vi "DAQ with LabVIEW 2.0.vi"() -> ()   [LabVIEW 2020]
uses:
  <vilib>/MakerHub/LINX/Public/Peripherals/Analog/Analog Read 1 Chan.vi
  <vilib>/MakerHub/LINX/Public/Peripherals/Digital/Digital Write 1 Chan.vi
  <vilib>/MakerHub/LINX/Public/Peripherals/Analog/Analog Read N Chans.vi
  <vilib>/MakerHub/LINX/Public/Peripherals/Digital/Digital Write N Chans.vi
  <vilib>/MakerHub/LINX/Private/Local IO/LinxAnalogRead.vi
  <vilib>/MakerHub/LINX/Public/Utilities/Check Channel.vi
  <vilib>/MakerHub/LINX/Private/Local IO/LinxDigitalWrite.vi
  <vilib>/MakerHub/LINX/Public/Utilities/Open Serial.vi
  <vilib>/MakerHub/LINX/Private/Utilties/Generate Error.vi
  <vilib>/MakerHub/LINX/LMH-LINX.lvlib
panel:
  out "String":string
  out "Vertical Graduated Bar":u8(slide) scale=0.0..60.0
  out "Gauge":dbl(knob) scale=0.0..10.0
  out "Voltage 5":dbl
  out "Voltage 4":dbl
  in  "FAN":bool
  out "LDR":dbl(graph)
  out "Loop Rate (Hz)":u32
  out "Voltage 3":dbl
  out "Voltage 2":dbl
  out "Voltage":dbl
  out "Soil Moisture":dbl(graph)
  out "MQ-135":dbl(graph)
  in  "Lights":bool
  in  "STOP":bool
  in  "COM PORT":refnum<visa-resource-name>="N/A"
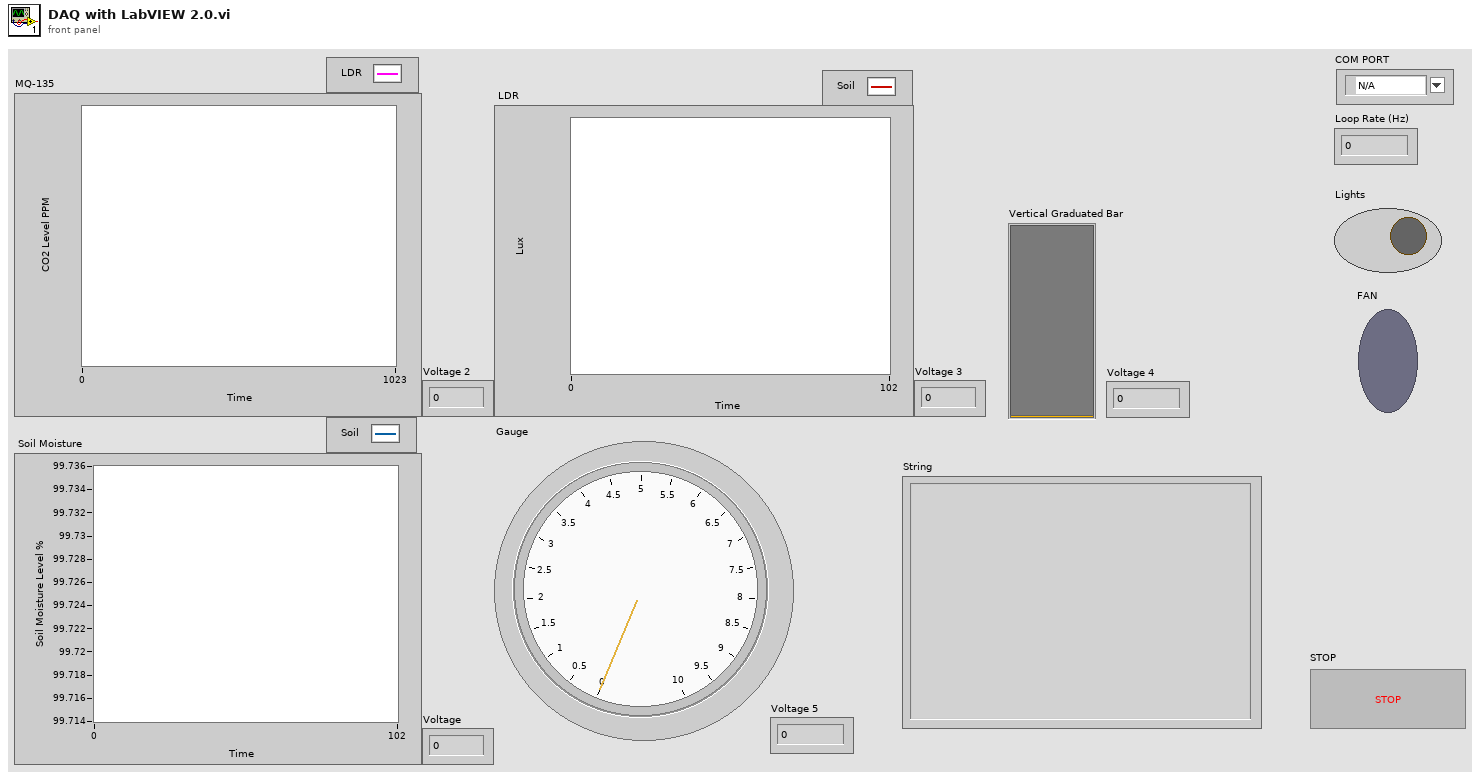
[diagram p1: front panel]
types:
  T1 = typedef "LMH-LINX.lvlib/LINX Ref.ctl" = cluster{"IO":T2, "Interface":T3, "LINX Device Config":T4}
  T2 = typedef "LMH-LINX.lvlib/Platform.ctl" = enum16{"Remote", "Local"}
  T3 = typedef "LMH-LINX.lvlib/Interface.ctl" = enum16{"Serial", "TCP"}
  T4 = typedef "LMH-LINX.lvlib/Device.lvlib/LINX Device Config.ctl" = cluster{"Interface":T3, "COM Port":refnum<visa-resource-name>, "TCP Configuration":T5, "Device Family":u8, "Device ID":u8, "Device Name":string, "TCP Ref":refnum<k5>, "Channels":T6}
  T5 = typedef "LMH-LINX.lvlib/Device.lvlib/TCP Config.ctl" = cluster{"IP Address":string, "Port":u16}
  T6 = typedef "LMH-LINX.lvlib/Channels.ctl" = cluster{"DI":u8[], "DO":u8[], "AI":u8[], "AO":u8[], "PWM":u8[], "QE":u8[], "UART":u8[], "I2C 2":u8[], "SPI":u8[], "CAN":u8[], "Servo":u8[], "AI Ref (V)":dbl, "AI Resolution (Bits)":u8, "AO Ref (V)":dbl, "AO Resolution (Bits)":u8}
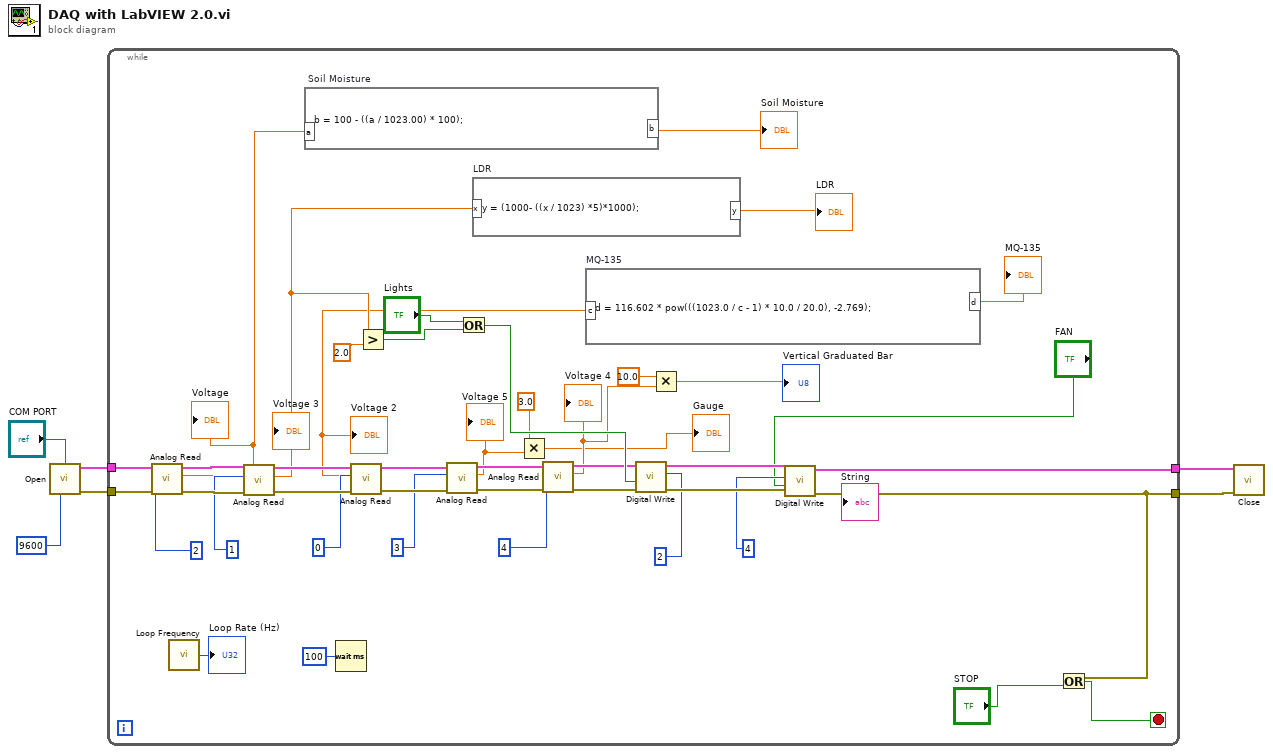
[diagram p0: block diagram]
diagram:
  n1 = call-poly <vilib>:"Open.vi"("Baud Rate Override"=u32 9600, "Serial Port"="COM PORT") -> ("Error Out"=w1:errorcluster, "LINX Resource"=w2:T1)  [unwired: 7 in, 1 out]
  n2 = while {
    tunnel: [w28] -> w4
    tunnel: [w27] -> w3
    tunnel: w2 -> [w37]
    tunnel: w1 -> [w36]
    stop <- w40 stop-if-true
    n3 = call-poly <vilib>:"Analog Read.vi"("Error In"=w36, "Analog Channel"=u8 2, "LINX Resource"=w37) -> ("Error Out"=w48:errorcluster, "Voltage"=w31:dbl, "LINX Resource"=w49:T1)  [unwired: 5 in, 1 out]
    "Voltage" <- w31
    n4 = call <vilib>:"Loop Frequency.vi"() -> ("Loop Rate (Hz)"=→"Loop Rate (Hz)":u32)
    n5 = call-poly <vilib>:"Analog Read.vi"("Error In"=w48, "Analog Channel"=u8 1, "LINX Resource"=w49) -> ("Error Out"=w46:errorcluster, "Voltage"=w34:dbl, "LINX Resource"=w47:T1)  [unwired: 5 in, 1 out]
    "Voltage 3" <- w34
    n6 = formula code="b = 100 - ((a / 1023.00) * 100);" "Soil Moisture"("a"=w31) -> ("b"=→"Soil Moisture":dbl)
    n7 = Wait (ms)(milliseconds to wait=u32 100) -> ()  [unwired: 1 out]
    n8 = call-poly <vilib>:"Analog Read.vi"("Error In"=w46, "Analog Channel"=u8 0, "LINX Resource"=w47) -> ("Error Out"=w19:errorcluster, "Voltage"=w32:dbl, "LINX Resource"=w20:T1)  [unwired: 5 in, 1 out]
    "Voltage 2" <- w32
    n9 = Greater?(x=w34, y=2.0) -> (0:w45:bool)
    n10 = call-poly <vilib>:"Analog Read.vi"("Error In"=w19, "Analog Channel"=u8 3, "LINX Resource"=w20) -> ("Error Out"=w17:errorcluster, "Voltage"=w9:dbl, "LINX Resource"=w18:T1)  [unwired: 5 in, 1 out]
    "Voltage 5" <- w9
    n11 = Or(x="Lights", y=w45) -> (x .or. y?=w22:bool)
    n12 = formula code="y = (1000- ((x / 1023) *5)*1000);" "LDR"("x"=w34) -> ("y"=→"LDR":dbl)
    n13 = Multiply(x=3.0, y=w9) -> (x*y=→"Gauge":dbl)
    n14 = call-poly <vilib>:"Analog Read.vi"("Error In"=w17, "Analog Channel"=u8 4, "LINX Resource"=w18) -> ("Error Out"=w13:errorcluster, "Voltage"=w12:dbl, "LINX Resource"=w14:T1)  [unwired: 5 in, 1 out]
    "Voltage 4" <- w12
    n15 = formula code="d = 116.602 * pow(((1023.0 / c - 1) * 10.0 / 20.0), -2.769);" "MQ-135"("c"=w32) -> ("d"=→"MQ-135":dbl)
    n16 = call-poly <vilib>:"Digital Write.vi"("Error In"=w13, "Output Value"=w22, "DO Channel"=u8 2 ("DI Channel"), "LINX Resource"=w14) -> ("Error Out"=w26:errorcluster, "LINX Resource"=w25:T1)  [unwired: 6 in]
    n17 = Multiply(x=10.0, y=w12) -> (x*y=→"Vertical Graduated Bar":dbl)
    n18 = call-poly <vilib>:"Digital Write.vi"("Error In"=w26, "Output Value"="FAN", "DO Channel"=u8 4, "LINX Resource"=w25) -> ("Error Out"=w27:errorcluster, "LINX Resource"=w28:T1)  [unwired: 6 in]
    n19 = Or(x=w27, y="STOP") -> (x .or. y?=w40:bool)
  }
  n20 = call <vilib>:"Close.vi"("Error In"=w3, "LINX Resource"=w4) -> ()  [unwired: 9 in, 1 out]
